vi "IDS_rt_enableAaf.vi"(8 "error in (no error)":errorcluster, 11 "deviceHandle":i32) -> (0 "error out":errorcluster, 3 "deviceHandle out":i32)   [LabVIEW 2016]
doc: "int IDS_DLL IDS_ecu_enable();"
panel:
  in  "window":i32
  in  "attenuation":i32
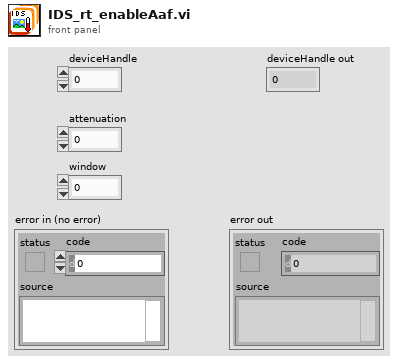
[diagram p1: front panel]
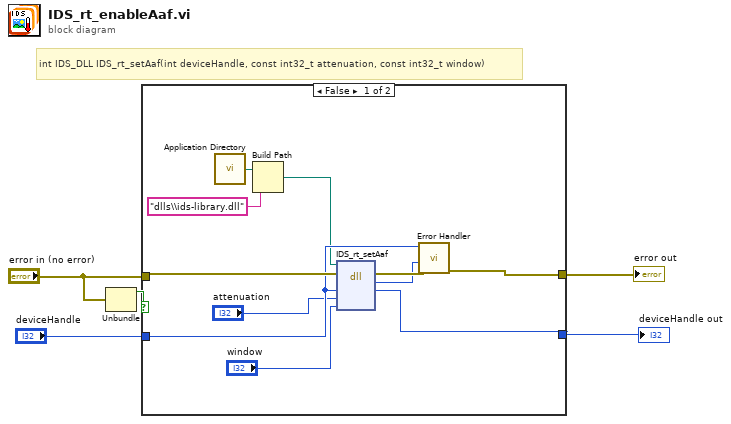
[diagram p0: block diagram]
diagram:
  # "int IDS_DLL IDS_rt_setAaf(int deviceHandle, const int32_t attenuation, const int32_t window)"
  n1 = Unbundle("error in (no error)") -> ("status"=w1:bool)  [unwired: 2 out]
  n2 = case shown="False" w1 {
    tunnel: "error in (no error)" -> [w16 w18]
    tunnel: [w14 w18] -> w5
    tunnel: "deviceHandle" -> [w12 w17]
    tunnel: [w13 w17] -> w3
    frame False {
      n3 = call <vilib>:"Application Directory.vi"() -> ("Application Directory"=w8:path)
      n4 = Build Path(base path=w8, name or relative path="dlls\\ids-library.dll" ("ipAddress")) -> (appended path=w6:path)
      n5 = dll-call lib="C:/Users/matheus/Desktop/LabVIEW_Draft_V1.6.0/dlls/ids-library.*" fn="IDS_rt_setAaf"(path in=w6, error in=w16, "deviceHandle"=w12, "attenuation"="attenuation", "window"="window") -> (error out=w15:errorcluster, "return type"=w11:i32, "deviceHandle"=w13:i32)  [unwired: 3 in, 1 out]
      n6 = call "Error Handler.vi"("error in (no error)"=w15, "error code"=w11, "deviceHandle"=w12) -> ("error out"=w14:errorcluster)  [unwired: 7 in, 1 out]
    }
    frame True {
    }
  }
  "error out" <- w5
  "deviceHandle out" <- w3
